vi "Gen - Data Path.vi"(8 "Error In":errorcluster) -> (0 "Error Out":errorcluster, 3 "Path":path)   [LabVIEW 2020]
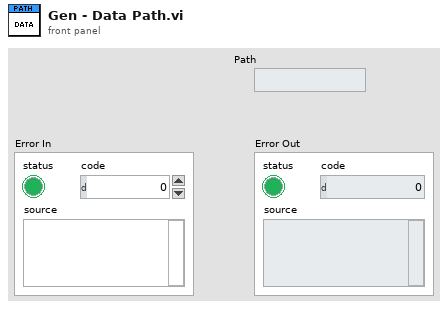
[diagram p1: front panel]
types:
  T1 = enum32{"invalid app kind", "Development System", "Run Time System", "Student Edition", "Embedded LabVIEW", "Evaluation", "Custom"}
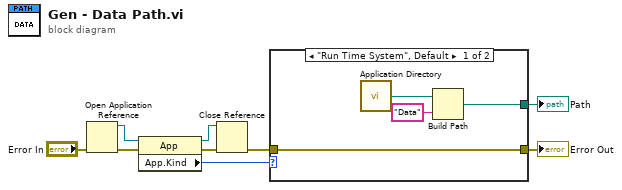
[diagram p0: block diagram]
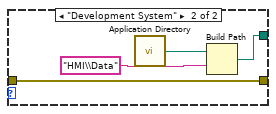
[diagram p2: hidden frame]
diagram:
  n1 = Open Application Reference(8:"Error In") -> (0:w9:errorcluster, 3:w4:refnum<vi>)  [unwired: 3 in]
  n2 = property class="App"(reference=w4, error in=w9) -> (reference out=w3:refnum<vi>, error out=w8:errorcluster, "App.Kind"=w2:T1)
  n3 = Close Reference(reference=w3, error in (no error)=w8) -> (error out=w7:errorcluster)
  n4 = case shown="\"Run Time System\", Default" w2 {
    tunnel: [w11 w15] -> w1
    tunnel: [w13 w17] -> w5
    tunnel: w7 -> [w13 w17]
    frame "Run Time System", Default {
      n5 = call <vilib>:"Application Directory.vi"() -> ("Application Directory"=w12:path)
      n6 = Build Path(base path=w12, name or relative path="Data") -> (appended path=w11:path)
    }
    frame "Development System" {
      n7 = call <vilib>:"Application Directory.vi"() -> ("Application Directory"=w16:path)
      n8 = Build Path(base path=w16, name or relative path="HMI\\Data") -> (appended path=w15:path)
    }
  }
  "Path" <- w1
  "Error Out" <- w5
